vi "Actor Core.vi"(8 "error in":errorcluster, 11 "Counter in":refnum<class "Counter.lvclass">) -> (0 "error out":errorcluster, 3 "Actor out":refnum<class "Actor.lvclass">)   [LabVIEW 2015, in "Counter.lvclass"]
doc: "(<B>Filename</B>: Actor Framework.lvlib:Actor.lvclass:Actor Core.vi)\n\nReceives messages to the actor, reacts to them, and initiates any error handling that may shut the actor down.\n\nDescendant classes may override this VI to append parallel tasks for the actor to complete while it handles messages. Overrides use the Call Parent Method node."
uses:
  Counter.lvclass
  <vilib>/ActorFramework/Actor/Actor.lvclass
  Counter Parameters.ctl
  Visa instrument/Visa instrument.lvclass
panel:
  in  "Parameters":T1={"Channels to measure"=[1]}
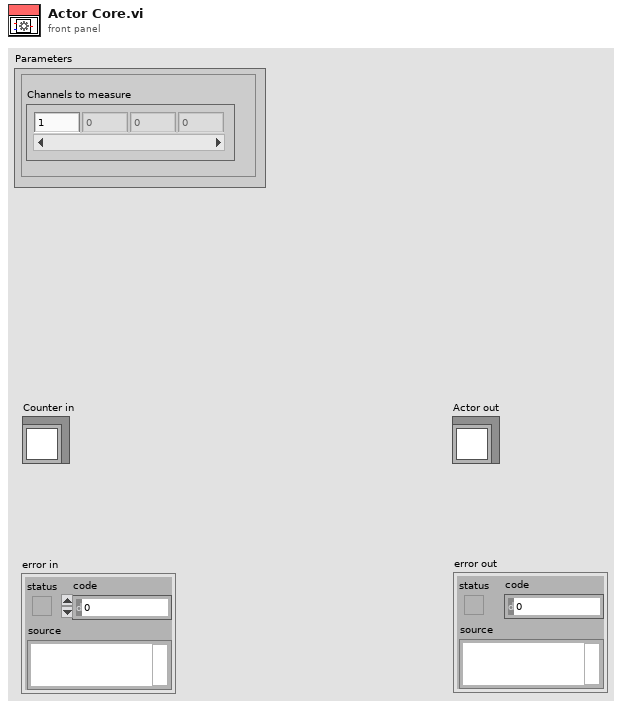
[diagram p1: front panel]
types:
  T1 = typedef "Counter Parameters.ctl" = cluster{"Channels to measure":i32[]}
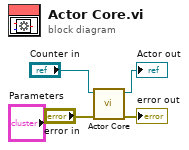
[diagram p0: block diagram]
diagram:
  n1 = call-parent "Actor Core.vi"("error in"="error in", "Mag Lab Measure Base in"="Counter in") -> ("error out"=→"error out":errorcluster, "Actor out"=→"Actor out":refnum<class "Actor.lvclass">)  [unwired: 8 in]
